vi "Idle_MakeCommandLaser.vi"(8 "Error In":errorcluster, 9 "Laser Control New":T1[](array[typedef])=[{"I Gain"=0.0, "D Gain"=0.0, "P Gain"=0.0, "Locking Tol."=0.0, "Wavelength "=0.0, "Temperature "=0.0, "Current "=0.0, "Detector Types"=enum."WV Online"}, {"I Gain"=0.0, "D Gain"=0.0, "P Gain"=0.0, "Locking Tol."=0.0, "Wavelength "=0.0, "Temperature "=0.0, "Current "=0.0, "Detector Types"=enum."WV Online"}, {"I Gain"=0.0, "D Gain"=0.0, "P Gain"=0.0, "Locking Tol."=0.0, "Wavelength "=0.0, "Temperature "=0.0, "Current "=0.0, "Detector Types"=enum."WV Online"}, {"I Gain"=0.0, "D Gain"=0.0, "P Gain"=0.0, "Locking Tol."=0.0, "Wavelength "=0.0, "Temperature "=0.0, "Current "=0.0, "Detector Types"=enum."WV Online"}, {"I Gain"=0.0, "D Gain"=0.0, "P Gain"=0.0, "Locking Tol."=0.0, "Wavelength "=0.0, "Temperature "=0.0, "Current "=0.0, "Detector Types"=enum."WV Online"}], 10 "Laser Control Old":T1[](array[typedef])=[{"I Gain"=0.0, "D Gain"=0.0, "P Gain"=0.0, "Locking Tol."=0.0, "Wavelength "=0.0, "Temperature "=0.0, "Current "=0.0, "Detector Types"=enum."WV Online"}, {"I Gain"=0.0, "D Gain"=0.0, "P Gain"=0.0, "Locking Tol."=0.0, "Wavelength "=0.0, "Temperature "=0.0, "Current "=0.0, "Detector Types"=enum."WV Online"}, {"I Gain"=0.0, "D Gain"=0.0, "P Gain"=0.0, "Locking Tol."=0.0, "Wavelength "=0.0, "Temperature "=0.0, "Current "=0.0, "Detector Types"=enum."WV Online"}, {"I Gain"=0.0, "D Gain"=0.0, "P Gain"=0.0, "Locking Tol."=0.0, "Wavelength "=0.0, "Temperature "=0.0, "Current "=0.0, "Detector Types"=enum."WV Online"}, {"I Gain"=0.0, "D Gain"=0.0, "P Gain"=0.0, "Locking Tol."=0.0, "Wavelength "=0.0, "Temperature "=0.0, "Current "=0.0, "Detector Types"=enum."WV Online"}], 11 "Queue In":refnum<queue>) -> (0 "Error Out":errorcluster, 1 "Laser Changed":i32=-1, 3 "Queue Out":refnum<queue>)   [LabVIEW 2012]
uses:
  TypeDef_LaserTypes.ctl
  TypeDef_LaserControl.ctl
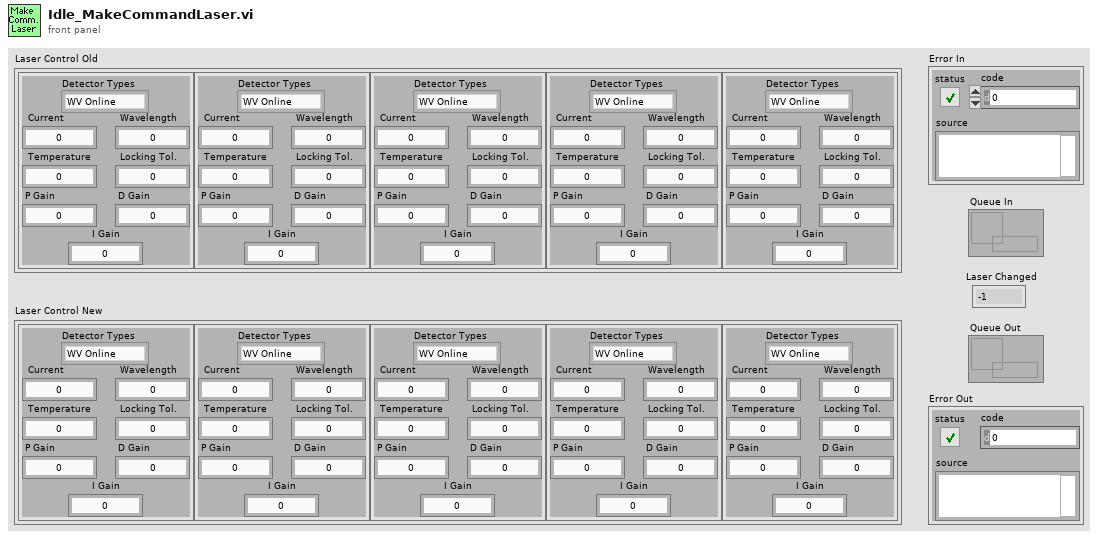
[diagram p1: front panel]
types:
  T1 = typedef "TypeDef_LaserControl.ctl" = cluster{"I Gain":dbl, "D Gain":dbl, "P Gain":dbl, "Locking Tol.":dbl, "Wavelength ":dbl, "Temperature ":dbl, "Current ":dbl, "Detector Types":T2}
  T2 = typedef "TypeDef_LaserTypes.ctl" = enum16{"WV Online", "WV Offline", "HSRL", "O2 Online", "O2 Offline"}
  T3 = cluster{"I Gain":bool, "D Gain":bool, "P Gain":bool, "Locking Tol.":bool, "Wavelength ":bool, "Temperature ":bool, "Current ":bool, "Detector Types":bool}[]
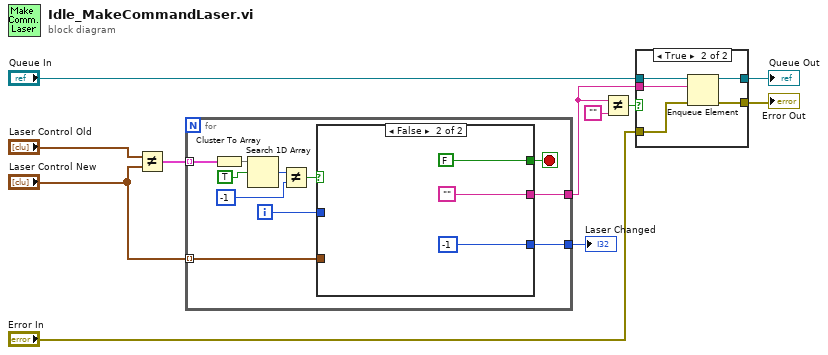
[diagram p0: block diagram]
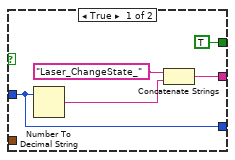
[diagram p3: hidden frame]
diagram:
  n1 = Not Equal?(x="Laser Control Old", y="Laser Control New") -> (x != y?=w11:T3)
  n2 = for {
    tunnel: w11 -> [w19] mode=indexing
    tunnel: "Laser Control New" -> [w15] mode=indexing
    tunnel: [w13] -> w10
    tunnel: [w12] -> w2
    i -> [w14]
    stop <- w17 stop-if-true
    n3 = Cluster To Array(cluster=w19) -> (array=w22:bool[])
    n4 = Search 1D Array(1D array=w22, element=TRUE) -> (index of element=w20:i32)  [unwired: 1 in]
    n5 = Not Equal?(x=w20, y=-1) -> (x != y?=w18:bool)
    n6 = case shown="False" w18 {
      tunnel: [TRUE FALSE] -> w17
      tunnel: w15 -> [_ _]
      tunnel: w14 -> [w24 _]
      tunnel: [w24 -1] -> w13
      tunnel: [w23 ""] -> w12
      frame True {
        n7 = Number To Decimal String(number=w24) -> (decimal integer string=w25:string)  [unwired: 1 in]
        n8 = Concatenate Strings("Laser_ChangeState_", w25) -> (w23:string)
      }
      frame False {
      }
    }
  }
  "Laser Changed" <- w10
  n9 = Not Equal?(x=w2, y="") -> (x != y?=w3:bool)
  n10 = case shown="True" w3 {
    tunnel: "Queue In" -> [w31 w37]
    tunnel: [w31 w36] -> w8
    tunnel: "Error In" -> [w32 w35]
    tunnel: [w32 w34] -> w6
    tunnel: w2 -> [_ w33]
    frame False {
    }
    frame True {
      n11 = Enqueue Element(queue=w37, element=w33, error in (no error)=w35) -> (queue out=w36:refnum<queue>, error out=w34:errorcluster)  [unwired: 1 in, 1 out]
    }
  }
  "Queue Out" <- w8
  "Error Out" <- w6
